vi "sg Close Device.vi"(8 "error in (no error)":errorcluster, 11 "device":i32) -> (0 "error out":errorcluster, 3 "function return":u32(ring))   [LabVIEW 2014, in "VSG25A.lvlib"]
doc: "SG_API sgStatus sgCloseDevice(int device);"
uses:
  VSG25A.lvlib
  sg_api.dll
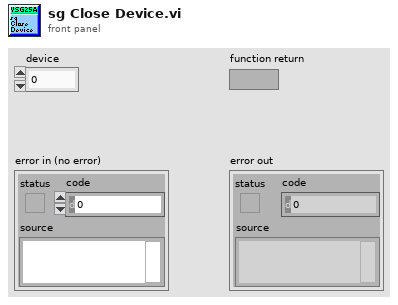
[diagram p1: front panel]
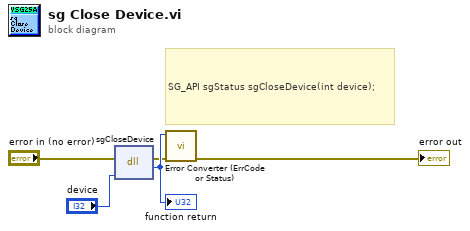
[diagram p0: block diagram]
diagram:
  # "SG_API sgStatus sgCloseDevice(int device);"
  n1 = dll-call lib="C:/Users/M_LAPTOP/Desktop/Labview/practice/VSG25A/sg_lib/sg_api.*" fn="sgCloseDevice"(error in="error in (no error)", "device"="device") -> (error out=w2:errorcluster, w5:u32)  [unwired: 3 in, 1 out]
  "function return" <- w5
  n2 = call "Error Converter (ErrCode or Status).vi"("error in (no error)"=w2, "error code"=w5) -> ("error out"=→"error out":errorcluster)  [unwired: 9 in]
